vi "ExWriteR3BFileHeader.vi"(0 "FileType":u32=67633152, 1 "Full File Name":path, 2 "Date/Time Start (Local)":string, 3 "error in (no error)":errorcluster, 4 "Date/Time Start (UTC)":string) -> (5 "error out":errorcluster)   [LabVIEW 2010]
panel:
  out "End Tic Count":u64
  out "Start Tic Count":u64
  in  "Date/Time End (UTC)":string
  in  "Date/Time End (Local)":string
  # "ExWriteR3BFileHeader.vi\nThis VI will use write information to the file header."
  # "File Types:\nSPE = 67371008\nTIF  = 67174400\nR3B = 67633152\nPMI = 67436544"
  # "Browse match pattern is set to *.r3b.  Modify this if different file type is needed."
  # "Date/Time MUST Be In This Format: mm-dd-yyyy hh:mm:ss"
  # "START"
  # "END"
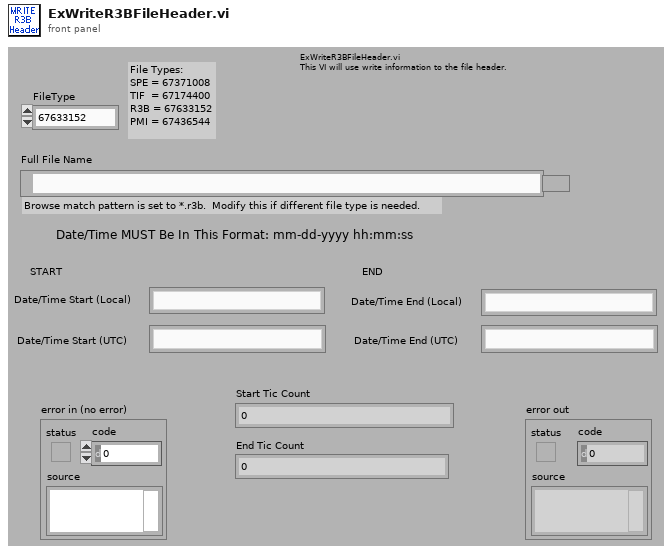
[diagram p1: front panel]
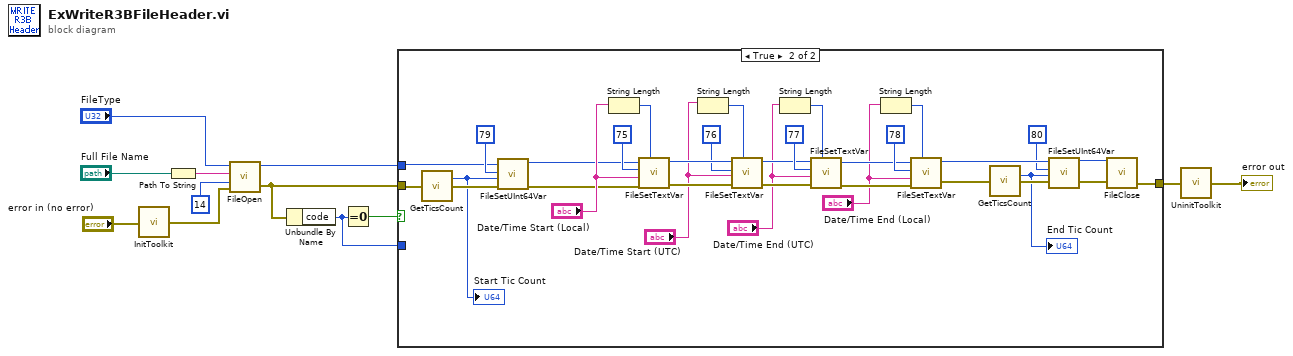
[diagram p0: block diagram]
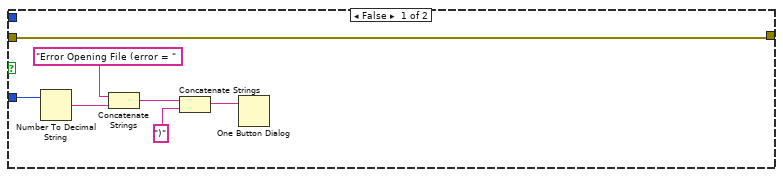
[diagram p2: hidden frame]
diagram:
  n1 = call <userlib>:"InitToolkit.vi"("error in"="error in (no error)") -> ("error out"=w3:errorcluster)
  n2 = Path To String(path="Full File Name") -> (string=w10:string)
  n3 = call <userlib>:"FileOpen.vi"("error in"=w3, "File Operations"=14, "FileName"=w10, "File Type"="FileType") -> ("error out"=w7:errorcluster, "File Handle"=w6:u32)
  n4 = Unbundle By Name(w7) -> ("code"=w5:i32)
  n5 = Equal To 0?(x=w5) -> (x = 0?=w8:bool)
  n6 = case shown="True" w8 {
    tunnel: w7 -> [w13 w47]
    tunnel: w6 -> [_ w31]
    tunnel: w5 -> [w19 _]
    tunnel: [w13 w48] -> w2
    frame False {
      n7 = Number To Decimal String(number=w19) -> (decimal integer string=w18:string)  [unwired: 1 in]
      n8 = Concatenate Strings("Error Opening File (error = ", w18) -> (w16:string)
      n9 = Concatenate Strings(w16, ")") -> (w14:string)
      n10 = One Button Dialog(message=w14) -> ()  [unwired: 1 in, 1 out]
    }
    frame True {
      n11 = call <userlib>:"GetTicsCount.vi"("error in"=w47) -> ("Tic Count"=w32:u64, "error out"=w35:errorcluster)
      "Start Tic Count" <- w32
      n12 = call <userlib>:"FileSetUInt64Var.vi"("error in"=w35, "Value"=w32, "Parameter ID"=79, "File Handle"=w31) -> ("error out"=w34:errorcluster, "File Handle"=w30:u32)
      n13 = String Length(string="Date/Time Start (Local)") -> (length=w45:i32)
      n14 = call <userlib>:"FileSetTextVar.vi"("File Handle"=w30, "Parameter ID"=75, "Text Value"="Date/Time Start (Local)", "error in"=w34, "Size Of Text Value"=w45) -> ("File Handle"=w50:u32, "error out"=w51:errorcluster)
      n15 = String Length(string="Date/Time Start (UTC)") -> (length=w43:i32)
      n16 = call <userlib>:"FileSetTextVar.vi"("File Handle"=w50, "Parameter ID"=76, "Text Value"="Date/Time Start (UTC)", "error in"=w51, "Size Of Text Value"=w43) -> ("File Handle"=w40:u32, "error out"=w38:errorcluster)
      n17 = String Length(string="Date/Time End (UTC)") -> (length=w22:i32)
      n18 = call <userlib>:"FileSetTextVar.vi"("File Handle"=w40, "Parameter ID"=77, "Text Value"="Date/Time End (UTC)", "error in"=w38, "Size Of Text Value"=w22) -> ("File Handle"=w39:u32, "error out"=w37:errorcluster)
      n19 = String Length(string="Date/Time End (Local)") -> (length=w21:i32)
      n20 = call <userlib>:"FileSetTextVar.vi"("File Handle"=w39, "Parameter ID"=78, "Text Value"="Date/Time End (Local)", "error in"=w37, "Size Of Text Value"=w21) -> ("File Handle"=w27:u32, "error out"=w36:errorcluster)
      n21 = call <userlib>:"GetTicsCount.vi"("error in"=w36) -> ("Tic Count"=w24:u64, "error out"=w29:errorcluster)
      "End Tic Count" <- w24
      n22 = call <userlib>:"FileSetUInt64Var.vi"("error in"=w29, "Value"=w24, "Parameter ID"=80, "File Handle"=w27) -> ("error out"=w28:errorcluster, "File Handle"=w26:u32)
      n23 = call <userlib>:"FileClose.vi"("error in"=w28, "File Handle"=w26) -> ("error out"=w48:errorcluster)
    }
  }
  n24 = call <userlib>:"UninitToolkit.vi"("error in"=w2) -> ("error out"=→"error out":errorcluster)
